vi "Write to File.vi"(7 "Column Header":string[][](array[string])=[["Time (Rel)", "Time (Abs)", "Pump Elapsed Time", "PS Voltage", "Controller Cmd", "Pump/Ctrl Voltage", "Pump Current", "Controller Current", "Target Speed", "Pump Speed", "Press/Flow Cmd", "Pump Pressure", "Pump Flow", "Tank 1 Temp Cmd", "Tank 1 Temp", "Tank 2 Temp Cmd", "Tank 2 Temp"], ["Hours", "Seconds", "Seconds", "Volts", "%", "Volts", "Amps", "Amps", "RPM", "RPM", "", "kPA", "LPH", "degC", "degC", "degC", "degC"]], 9 "Filename":string, 10 "Data":string[](array[string]), 11 "Path":path) -> ()   [LabVIEW 2019]
uses:
  <vilib>/Utility/file.llb/Write To Spreadsheet File (string).vi
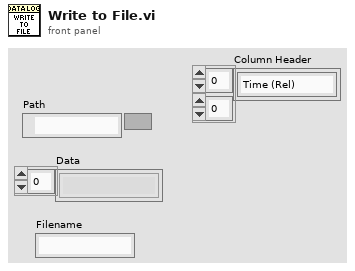
[diagram p1: front panel]
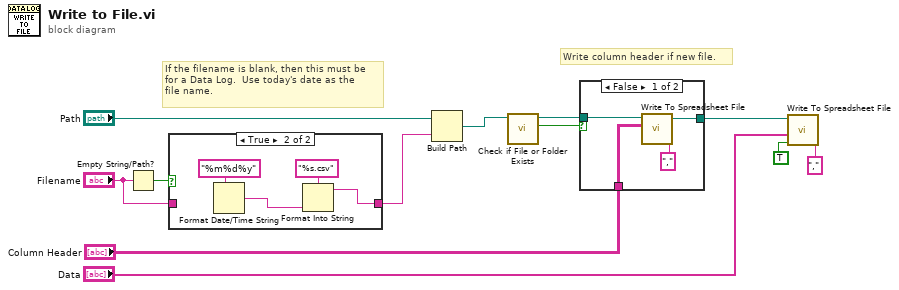
[diagram p0: block diagram]
diagram:
  # "If the filename is blank, then this must be\nfor a Data Log.  Use today's date as the\nfile name."
  # "Write column header if new file."
  n1 = Empty String/Path?(string/path="Filename") -> (empty?=w4:bool)
  n2 = case shown="True" w4 {
    tunnel: "Filename" -> [w13 _]
    tunnel: [w13 w14] -> w2
    frame False {
    }
    frame True {
      n3 = Format Date/Time String(time format string (%c)="%m%d%y") -> (date/time string=w16:string)  [unwired: 2 in]
      n4 = Format Into String(format string="%s.csv", w16) -> (resulting string=w14:string)  [unwired: 2 in, 1 out]
    }
  }
  n5 = Build Path(base path="Path", name or relative path=w2) -> (appended path=w5:path)
  n6 = call <vilib>:"Check if File or Folder Exists.vi"("path"=w5) -> ("file or folder exists?"=w12:bool, "dup path"=w11:path)  [unwired: 8 in, 1 out]
  n7 = case shown="False" w12 {
    tunnel: w11 -> [w21 w22]
    tunnel: "Column Header" -> [w20 _]
    tunnel: [w19 w22] -> w9
    frame False {
      n8 = call-poly <vilib>:"Write To Spreadsheet File.vi"("delimiter (\\t)"="," ("delimiter (\\t)"), "2D data"=w20, "file path (dialog if empty)"=w21) -> ("new file path (Not A Path if cancelled)"=w19:path)  [unwired: 5 in]
    }
    frame True {
    }
  }
  n9 = call-poly <vilib>:"Write To Spreadsheet File.vi"("delimiter (\\t)"="," ("delimiter (\\t)"), "append to file? (new file:F)"=TRUE, "1D data"="Data", "file path (dialog if empty)"=w9) -> ()  [unwired: 4 in, 1 out]
